vi "Get NEW FI Set Max.vi"(8 "error in (no error)":errorcluster) -> (0 "Error Out":errorcluster, 1 "Get Max_Out":dbl)   [LabVIEW 2023]
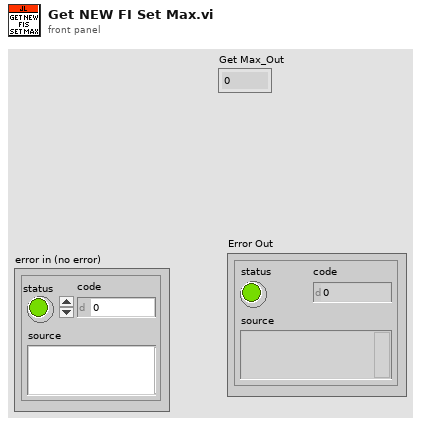
[diagram p1: front panel]
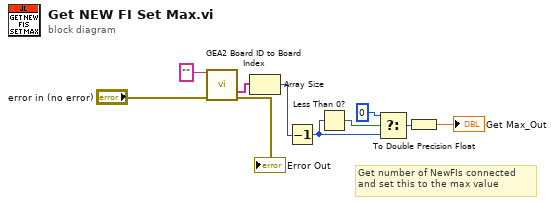
[diagram p0: block diagram]
diagram:
  # "Get number of NewFIs connected\nand set this to the max value"
  n1 = call "GEA2 Board ID to Board Index.vi"("Board ID"="", "Error In"="error in (no error)") -> ("Boards Found"=w9:string[], "Error Out"=→"Error Out":errorcluster)  [unwired: 9 in, 3 out]
  n2 = Array Size(array=w9) -> (size(s)=w4:i32)
  n3 = Decrement(x=w4) -> (x-1=w6:i32)
  n4 = Less Than 0?(x=w6) -> (x < 0?=w5:bool)
  n5 = Select(t=0, s=w5, f=w6) -> (s? t:f=w8:i32)
  n6 = To Double Precision Float(number=w8) -> (double precision float=→"Get Max_Out":dbl)
